vi "ReadBaseTime.vi"(6 "文件时间？(F)":bool, 7 "时间字符":string, 8 "日期字符":string) -> (2 "基时间簇":T1)   [LabVIEW 2015]
uses:
  <vilib>/Utility/miscctls.llb/LVDateTimeRec.ctl
  <vilib>/regexp/Match Regular Expression.xnode
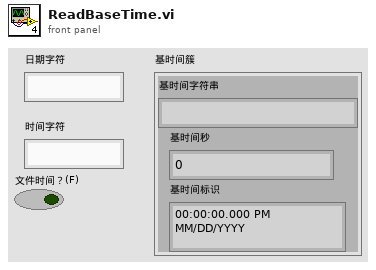
[diagram p1: front panel]
types:
  T1 = cluster{"基时间字符串":string, "基时间秒":dbl, "基时间标识":timestamp}
  T2 = typedef "LVDateTimeRec.ctl" = cluster{"fractional second":dbl, "second":i32, "minute":i32, "hour":i32, "day of month":i32, "month":i32, "year":i32, "day of week":i32, "day of year":i32, "DST":i32}
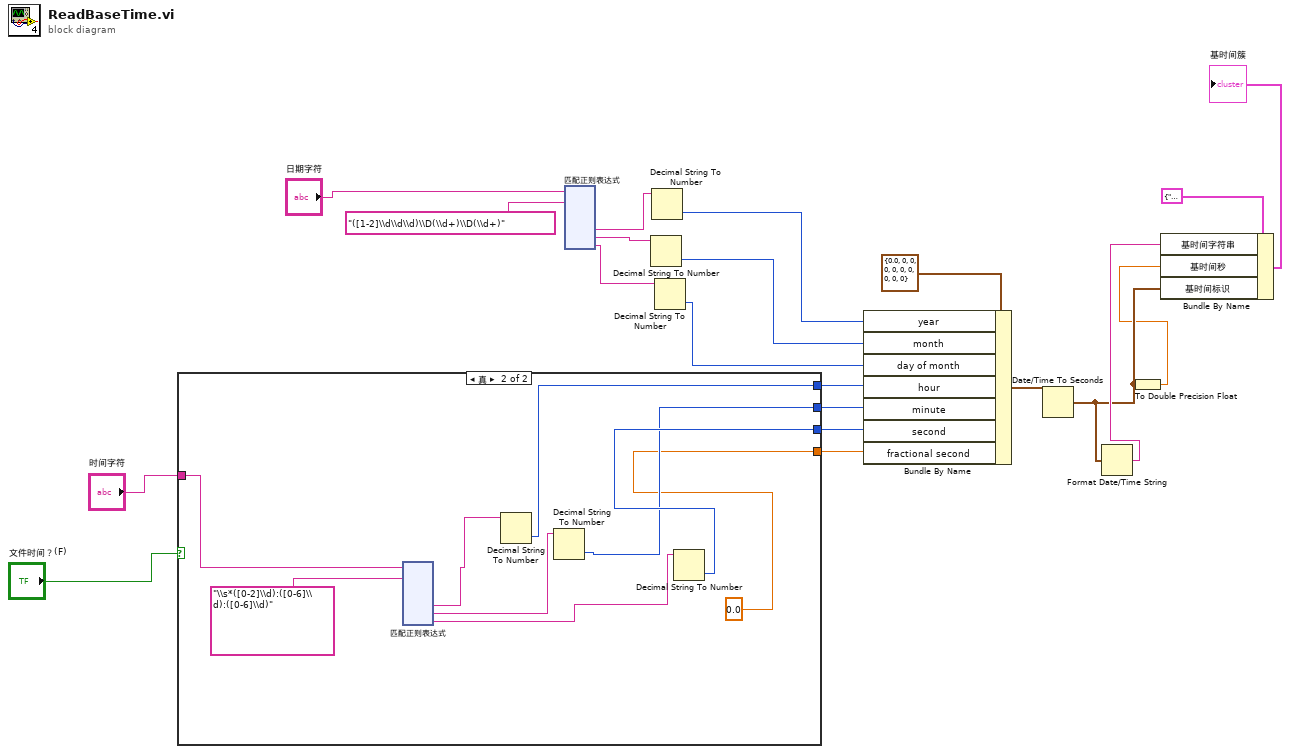
[diagram p0: block diagram]
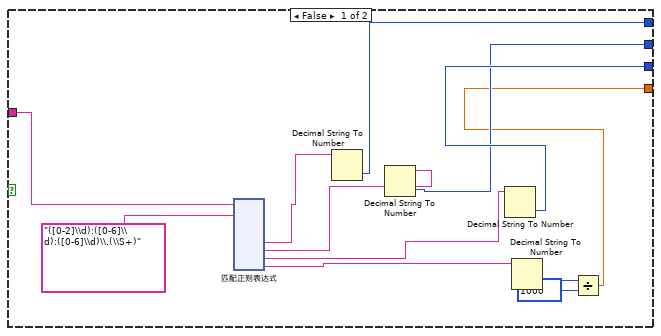
[diagram p2: hidden frame]
diagram:
  n1 = case shown="真" "文件时间？(F)" {
    tunnel: [w22 0.0] -> w21
    tunnel: [w33 w161] -> w20
    tunnel: [w32 w160] -> w19
    tunnel: [w31 w159] -> w18
    tunnel: "时间字符" -> [w23 w154]
    frame False {
      n2 = xnode "匹配正则表达式"("输入字符串"=w23, "正则表达式"="([0-2]\\d):([0-6]\\d):([0-6]\\d)\\.(\\S+)") -> ("子匹配 1"=w25:string, "子匹配 2"=w26:string, "子匹配 3"=w27:string, "子匹配 4"=w29:string)  [unwired: 4 in, 5 out]
      n3 = Decimal String To Number(string=w25) -> (number=w31:i32)  [unwired: 2 in, 1 out]
      n4 = Decimal String To Number(string=w26) -> (number=w32:i32)  [unwired: 2 in, 1 out]
      n5 = Decimal String To Number(string=w27) -> (number=w33:i32)  [unwired: 2 in, 1 out]
      n6 = Decimal String To Number(string=w29) -> (number=w28:i32)  [unwired: 2 in, 1 out]
      n7 = Divide(x=w28, y=1000) -> (x/y=w22:dbl)
    }
    frame True {
      n8 = xnode "匹配正则表达式"("输入字符串"=w154, "正则表达式"="\\s*([0-2]\\d):([0-6]\\d):([0-6]\\d)") -> ("子匹配 1"=w156:string, "子匹配 2"=w157:string, "子匹配 3"=w158:string)  [unwired: 4 in, 5 out]
      n9 = Decimal String To Number(string=w156) -> (number=w159:i32)  [unwired: 2 in, 1 out]
      n10 = Decimal String To Number(string=w157) -> (number=w160:i32)  [unwired: 2 in, 1 out]
      n11 = Decimal String To Number(string=w158) -> (number=w161:i32)  [unwired: 2 in, 1 out]
    }
  }
  n12 = xnode "匹配正则表达式"("输入字符串"="日期字符", "正则表达式"="([1-2]\\d\\d\\d)\\D(\\d+)\\D(\\d+)") -> ("子匹配 1"=w8:string, "子匹配 2"=w7:string, "子匹配 3"=w6:string)  [unwired: 4 in, 5 out]
  n13 = Decimal String To Number(string=w7) -> (number=w16:i32)  [unwired: 2 in, 1 out]
  n14 = Decimal String To Number(string=w8) -> (number=w15:i32)  [unwired: 2 in, 1 out]
  n15 = Decimal String To Number(string=w6) -> (number=w17:i32)  [unwired: 2 in, 1 out]
  n16 = Bundle By Name(cluster=T2 {"fractional second"=0.0, "second"=0, "minute"=0, "hour"=0, "day of month"=0, "month"=0, "year"=0, "day of week"=0, "day of year"=0, "DST"=0} ("日期时间记录"), "year"=w15, "month"=w16, "day of month"=w17, "hour"=w18, "minute"=w19, "second"=w20, "fractional second"=w21) -> (w3:T2)
  n17 = Date/Time To Seconds(2:w3) -> (0:w12:timestamp)  [unwired: 1 in]
  n18 = Format Date/Time String(seconds (now)=w12) -> (date/time string=w13:string)  [unwired: 2 in]
  n19 = To Double Precision Float(number=w12) -> (double precision float=w11:dbl)
  n20 = Bundle By Name(cluster=T1 {"基时间字符串"="", "基时间秒"=0.0, "基时间标识"=timestamp(0 s since 1904-01-01)} ("基时间簇"), "基时间字符串"=w13, "基时间秒"=w11, "基时间标识"=w12) -> (→"基时间簇":T1)
